vi "Drive.vi"(7 "Enum":T1, 8 "error in (no error)":errorcluster, 9 "Right":dbl, 10 "Left":dbl, 11 "MotorName":string="TankDrive") -> (0 "error out":errorcluster)   [LabVIEW 2013]
uses:
  TankDriveEnum.ctl
  <vilib>/Rock Robotics/WPI/RobotDrive/WPI_RobotDriveGetSetRefNum.vi
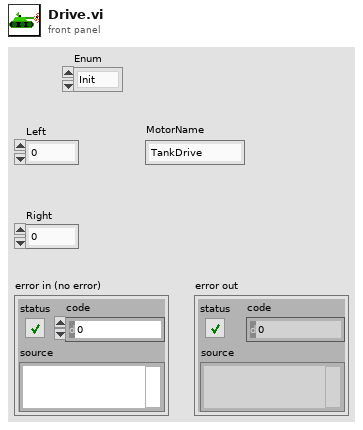
[diagram p1: front panel]
types:
  T1 = typedef "TankDriveEnum.ctl" = enum16{"Init", "SetValue", "Disable", "Linear Drive"}
  T2 = typedef "WPI_RobotDriveDevRef.ctl" = cluster{"DevStatus":errorcluster, "Motors[]":T3[], "Square Inputs":bool, "Max Output":dbl, "Isochronous":bool}
  T3 = typedef "WPI_MotorControlDeviceRef.ctl" = cluster{"DeviceStatus":errorcluster, "Type":enum16{"PWM", "CAN"}, "PWM":cluster{"Digital Module":T4, "PWM Channel":T5, "DeadBand":T6}, "CAN":cluster{"Device Number":u8, "Control Mode":T7, "Semaphore":T8, "Max Vout":dbl}, "Invert":bool, "TransformRef":T9, "InvTransformRef":T9}
  T4 = typedef "FPGA_TypedefDigitalModule.ctl" = enum16{"Digital Module 1", "Digital Module 2"}
  T5 = typedef "FPGA_DIOPWMChannel.ctl" = enum8{"PWM 1", "PWM 2", "PWM 3", "PWM 4", "PWM 5", "PWM 6", "PWM 7", "PWM 8", "PWM 9", "PWM 10", "Invalid"}
  T6 = typedef "WPI_PWMDeadband.ctl" = cluster{"Name":string, "maxPositivePwm":i32, "minPositivePwm":i32, "centerPwm":i32, "maxNegativePwm":i32, "minNegativePwm":i32, "angularRange":u16}
  T7 = typedef "WPI_CANJaguar_ControlMode.ctl" = enum8{"Percent VBus", "Current", "Speed", "Position", "Voltage"}
  T8 = typedef "Semaphore RefNum" = refnum<k1>
  T9 = typedef "WPI_PWMTransform_ConPane.ctl" = refnum<vi>
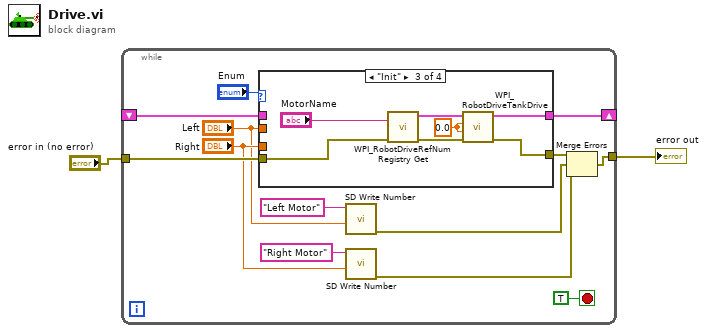
[diagram p0: block diagram]
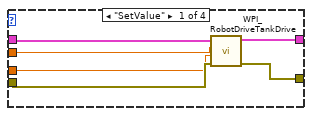
[diagram p2: hidden frame]
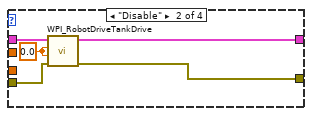
[diagram p3: hidden frame]
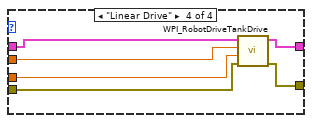
[diagram p4: hidden frame]
diagram:
  n1 = while {
    shift-right: [w15] -> _
    shift-left: _ -> [w13]
    tunnel: [w4] -> w2
    tunnel: "error in (no error)" -> [w11]
    stop <- TRUE stop-if-true
    n2 = case shown="\"Init\"" "Enum" {
      tunnel: [w20 w25 w32 w37] -> w15
      tunnel: w13 -> [w21 w26 _ w36]
      tunnel: w11 -> [w19 w23 w30 w39]
      tunnel: [w18 w22 w28 w38] -> w5
      tunnel: "Left" -> [w17 _ _ w35]
      tunnel: "Right" -> [w16 _ _ w34]
      frame "SetValue" {
        n3 = call <vilib>:"WPI_RobotDriveTankDrive.vi"("error in (no error)"=w19, "Right axis value"=w16, "Left axis value"=w17, "RobotDriveDevRef"=w21) -> ("error out"=w18:errorcluster, "RobotDriveDevRef"=w20:T2)  [unwired: 5 in, 1 out]
      }
      frame "Disable" {
        w24 = 0.0
        n4 = call <vilib>:"WPI_RobotDriveTankDrive.vi"("error in (no error)"=w23, "Right axis value"=w24, "Left axis value"=w24, "RobotDriveDevRef"=w26) -> ("error out"=w22:errorcluster, "RobotDriveDevRef"=w25:T2)  [unwired: 5 in, 1 out]
      }
      frame "Init" {
        w31 = 0.0
        n5 = call <vilib>:"WPI_RobotDriveRefNum Registry Get.vi"("error in (no error)"=w30, "refnum name"="MotorName") -> ("error out"=w29:errorcluster, "RobotDriveDevRef"=w33:T2)  [unwired: 8 in]
        n6 = call <vilib>:"WPI_RobotDriveTankDrive.vi"("error in (no error)"=w29, "Right axis value"=w31, "Left axis value"=w31, "RobotDriveDevRef"=w33) -> ("error out"=w28:errorcluster, "RobotDriveDevRef"=w32:T2)  [unwired: 5 in, 1 out]
      }
      frame "Linear Drive" {
        n7 = call <vilib>:"WPI_RobotDriveTankDrive.vi"("error in (no error)"=w39, "Right axis value"=w34, "Left axis value"=w35, "RobotDriveDevRef"=w36) -> ("error out"=w38:errorcluster, "RobotDriveDevRef"=w37:T2)  [unwired: 5 in, 1 out]
      }
    }
    n8 = call <vilib>:"SD Write Number.vi"("Numeric"="Left", "Name"="Left Motor") -> ("error out"=w6:errorcluster)  [unwired: 8 in, 1 out]
    n9 = call <vilib>:"SD Write Number.vi"("Numeric"="Right", "Name"="Right Motor") -> ("error out"=w3:errorcluster)  [unwired: 8 in, 1 out]
    n10 = Merge Errors(w5, w6, w3) -> (w4:errorcluster)
  }
  "error out" <- w2
